vi "Update Waveform.vi"(8 "error in (no error)":errorcluster, 11 "Triangle in":refnum<class "Triangle.lvclass">) -> (0 "error out":errorcluster, 3 "Triangle out":refnum<class "Triangle.lvclass">)   [LabVIEW 2014, in "Triangle.lvclass"]
uses:
  Triangle.lvclass
  Waveform/Waveform.lvclass/Waveform.ctl
  <vilib>/measure/NI_MABase.lvlib
  Waveform/Waveform.lvclass
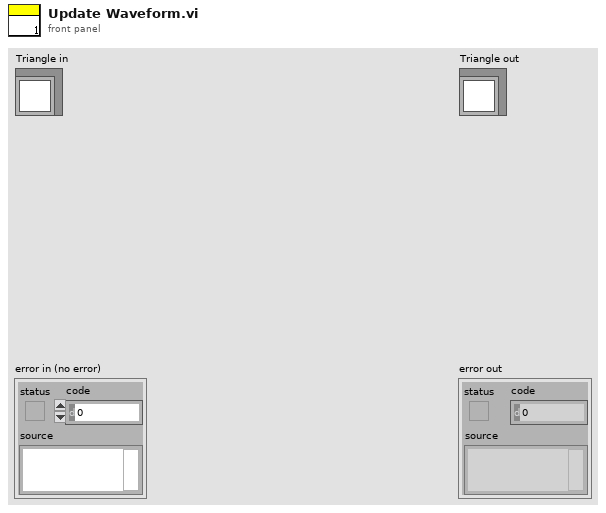
[diagram p1: front panel]
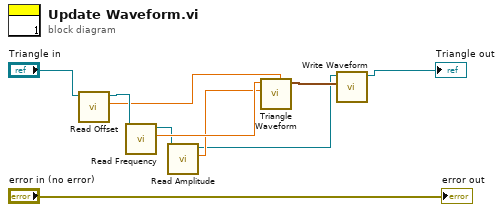
[diagram p0: block diagram]
diagram:
  n1 = call "Read Offset.vi"("Waveform in"="Triangle in") -> ("Offset"=w6:dbl, "Waveform out"=w7:refnum<class "Triangle.lvclass">)  [unwired: 8 in, 1 out]
  n2 = call "Read Frequency.vi"("Waveform in"=w7) -> ("Frequency"=w5:dbl, "Waveform out"=w3:refnum<class "Triangle.lvclass">)  [unwired: 8 in, 1 out]
  n3 = call "Read Amplitude.vi"("Waveform in"=w3) -> ("Amplitude"=w4:dbl, "Waveform out"=w1:refnum<class "Triangle.lvclass">)  [unwired: 8 in, 1 out]
  n4 = call <vilib>:"Triangle Waveform.vi"("offset"=w6, "amplitude"=w4, "frequency"=w5) -> ("signal out"=w9:waveform(dbl))  [unwired: 7 in, 1 out]
  n5 = call "Write Waveform.vi"("Waveform"=w9, "Waveform in"=w1) -> ("Waveform out"=→"Triangle out":refnum<class "Triangle.lvclass">)  [unwired: 8 in, 1 out]
  "error out" <- "error in (no error)"
